vi "Read Handler.vi"(8 "error in (no error)":errorcluster, 11 "Handler in":refnum<class "Handler.lvclass">) -> (0 "error out":errorcluster, 2 "Handler":refnum<k38>, 3 "Handler out":refnum<class "Handler.lvclass">)   [LabVIEW 2022 SP3, in "Logger.lvlib" / "Handler.lvclass"]
uses:
  Handler.lvclass
  Handler.lvclass/Handler.ctl
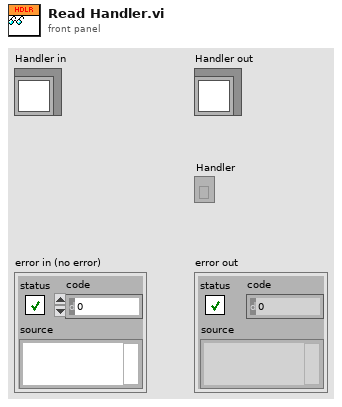
[diagram p1: front panel]
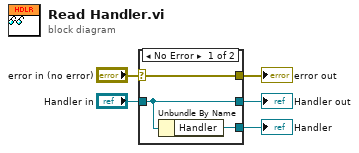
[diagram p0: block diagram]
diagram:
  n1 = case shown="No Error" "error in (no error)" {
    selector: "error in (no error)" -> [w8 w9]
    tunnel: [w8 w9] -> w4
    tunnel: [w7 w10] -> w2
    tunnel: "Handler in" -> [w7 w10]
    tunnel: [w6 _] -> w1
    frame No Error {
      n2 = Unbundle By Name(w7) -> ("Handler"=w6:refnum<k38>)
    }
    frame Error {
    }
  }
  "error out" <- w4
  "Handler out" <- w2
  "Handler" <- w1
